vi "Variable Z Script.vi"() -> ()   [LabVIEW 2010]
panel:
  in  "Strain Points":T1
  in  "Strain Directory":path=path "D:/Ab-initio/VASP Calcs/2D_Grain Boundaries/Batch25_20130914"
  in  "Structure Name":string="A3B12_Lamallar"
  in  "Structure File":path=path "D:/Ab-initio/VASP Calcs/2D_Grain Boundaries/Batch18_20130828/A3B12_Periodic_Twin/CONTCAR"
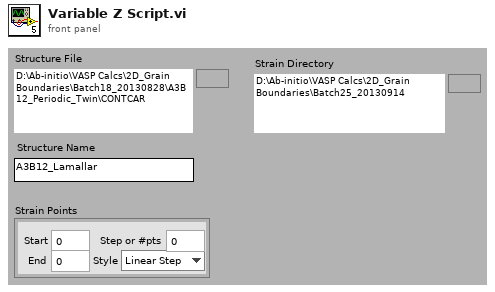
[diagram p1: front panel]
types:
  T1 = cluster{"Start":dbl, "End":dbl, "Step or #pts":dbl, "Style":enum16{"Linear Step", "Linear Pts", "Log Pts"}}
  T2 = cluster{"Structure Name":string, "Lattice vector a":dbl[], "Lattice vector b":dbl[], "Lattice vector c":dbl[], "Atoms Array":cluster{"Atom Name":string, "Positions (Direct)":dbl[][], "Positions (Cartesian)":dbl[][]}[], "# of atoms":i32}
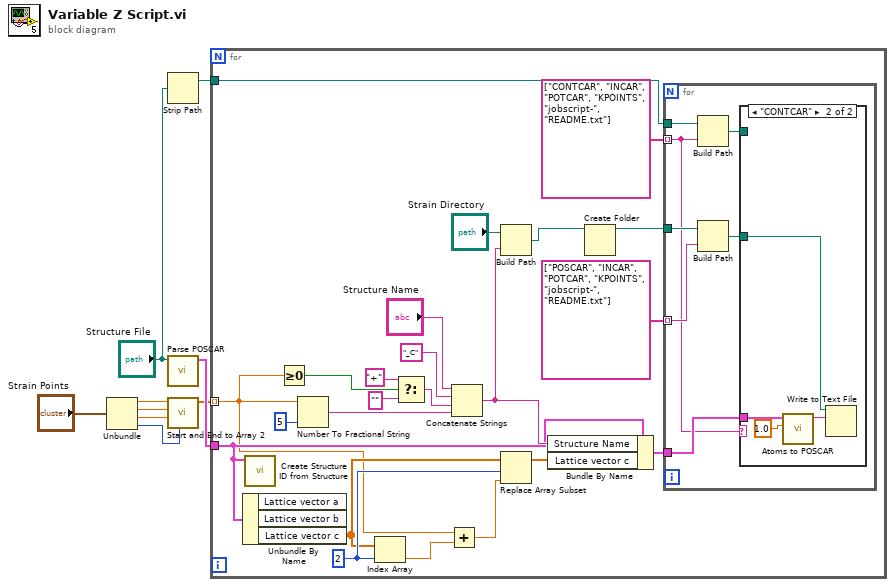
[diagram p0: block diagram]
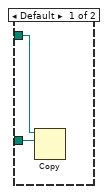
[diagram p2: hidden frame]
diagram:
  n1 = Unbundle("Strain Points") -> ("Start"=w7:dbl, "End"=w6:dbl, "Step or #pts"=w5:dbl, "Style"=w4:enum16{"Linear Step", "Linear Pts", "Log Pts"})
  n2 = Strip Path(path="Structure File") -> (stripped path=w1:path)  [unwired: 1 out]
  n3 = call "Parse POSCAR.vi"("POSCAR File"="Structure File") -> ("Structure"=w9:T2)  [unwired: 7 in, 3 out]
  n4 = call "Start and End to Array 2.vi"("Sweep Style"=w4, "Step or # Pts"=w5, "End"=w6, "Start"=w7) -> ("Array"=w3:dbl[])  [unwired: 7 in]
  n5 = for {
    tunnel: w9 -> [w23]
    tunnel: w3 -> [w22] mode=indexing
    tunnel: w1 -> [w13]
    w28 = 2 ("index")
    n6 = Unbundle By Name(w23) -> ("Lattice vector c"=w26:dbl[])  [unwired: 2 out]
    n7 = call "Create Structure ID from Structure.vi"("Structure"=w23) -> ()  [unwired: 10 in, 1 out]
    n8 = Greater Or Equal To 0?(x=w22) -> (x >= 0?=w21:bool)
    n9 = Number To Fractional String(number=w22, precision (6)=i16 5) -> (F-format string=w17:string)  [unwired: 2 in]
    n10 = Index Array(array=w26, index=w28) -> (element=w30:dbl)
    n11 = Select(t="+" ("string"), s=w21, f="") -> (s? t:f=w18:string)
    n12 = Add(x=w22, y=w30) -> (x+y=w29:dbl)
    n13 = Concatenate Strings("Structure Name", "_C" ("string"), w18, w17) -> (w24:string)
    n14 = Build Path(base path="Strain Directory", name or relative path=w24) -> (appended path=w10:path)
    n15 = Replace Array Subset(array=w26, new element=w29, index=w28) -> (w27:dbl[])
    n16 = Bundle By Name(cluster=w23, "Structure Name"=w24, "Lattice vector c"=w27) -> (w12:T2)
    n17 = Create Folder(path (use dialog)=w10) -> (created path=w14:path)  [unwired: 2 in, 2 out]
    n18 = for {
      tunnel: w13 -> [w39]
      tunnel: w14 -> [w37]
      tunnel: string[] ["CONTCAR", "INCAR", "POTCAR", "KPOINTS", "jobscript-", "README.txt"] -> [w33] mode=indexing
      tunnel: string[] ["POSCAR", "INCAR", "POTCAR", "KPOINTS", "jobscript-", "README.txt"] -> [w35] mode=indexing
      tunnel: w12 -> [w34]
      n19 = Build Path(base path=w39, name or relative path=w33) -> (appended path=w38:path)
      n20 = Build Path(base path=w37, name or relative path=w35) -> (appended path=w36:path)
      n21 = case shown="\"CONTCAR\"" w33 {
        tunnel: w38 -> [w41 _]
        tunnel: w36 -> [w40 w42]
        tunnel: w34 -> [_ w44]
        frame Default {
          n22 = Copy(10:w40, 11:w41) -> ()  [unwired: 3 in, 3 out]
        }
        frame "CONTCAR" {
          n23 = call "Atoms to POSCAR.vi"("Volume Factor"=1.0, "Atomic Structure"=w44) -> ("POSCAR File"=w45:string)  [unwired: 9 in]
          n24 = Write to Text File(file (use dialog)=w42, text=w45) -> ()  [unwired: 2 in, 3 out]
        }
      }
    }
  }
